vi "Should Read Body.vi"(8 "error in (no error)":errorcluster, 11 "Request in":refnum<class "Request.lvclass">) -> (0 "error out":errorcluster, 2 "Read Body?":bool, 3 "Request out":refnum<class "Request.lvclass">)   [LabVIEW 2023, in "Request.lvclass"]
doc: "Determines whether or not the Request should read a body, based on the Headers from the Client."
uses:
  Request.lvclass
  Request.lvclass/Request.ctl
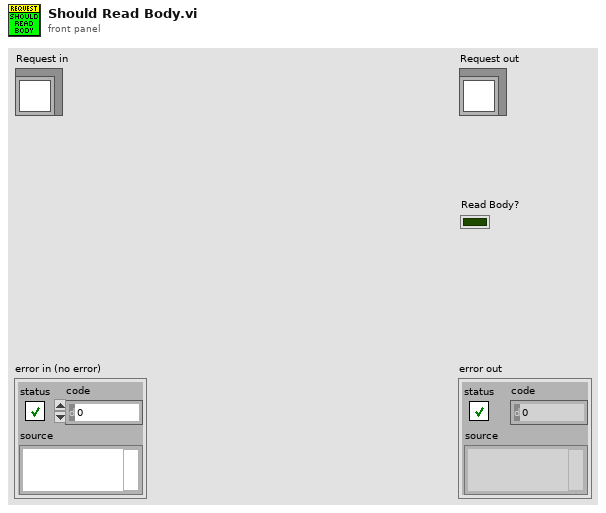
[diagram p1: front panel]
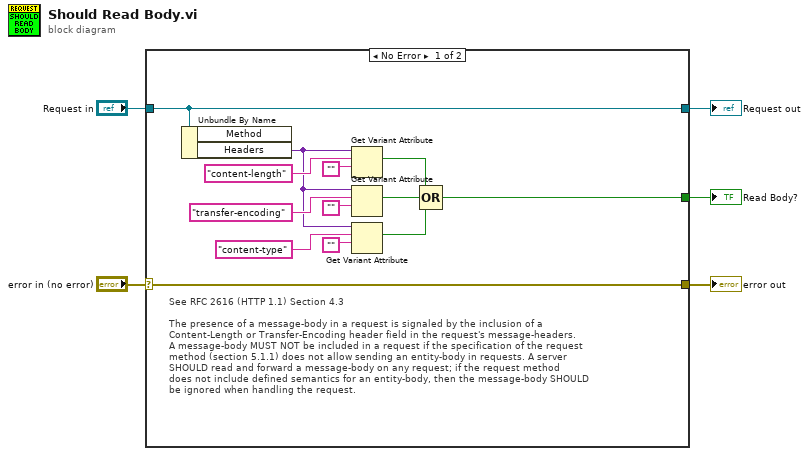
[diagram p0: block diagram]
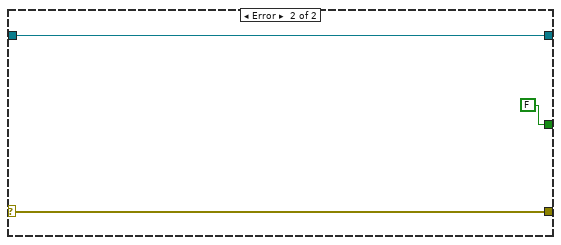
[diagram p2: hidden frame]
diagram:
  n1 = case shown="No Error" "error in (no error)" {
    selector: "error in (no error)" -> [w18 w21]
    tunnel: [w18 w21] -> w4
    tunnel: [w17 w20] -> w2
    tunnel: "Request in" -> [w17 w20]
    tunnel: [w11 FALSE] -> w1
    frame No Error {
      # "See RFC 2616 (HTTP 1.1) Section 4.3\n\nThe presence of a message-body in a request is signaled by the inclusion of a \nContent-Length or Transfer-Encoding header field in the request's message-headers. \nA message-body MUST NOT be included in a request if the specification of the request \nmethod (section 5.1.1) does not allow sending an entity-body in requests. A server \nSHOULD read and forward a message-body on any request; if the request method \ndoes not include defined semantics for an entity-body, then the message-body SHOULD \nbe ignored when handling the request."
      n2 = Unbundle By Name(w17) -> ("Headers"=w8:variant)  [unwired: 1 out]
      n3 = Get Variant Attribute(Variant=w8, name="content-length", default value (empty Variant)="") -> (found=w12:bool)  [unwired: 1 in, 3 out]
      n4 = Get Variant Attribute(Variant=w8, name="transfer-encoding", default value (empty Variant)="") -> (found=w7:bool)  [unwired: 1 in, 3 out]
      n5 = Get Variant Attribute(Variant=w8, name="content-type", default value (empty Variant)="") -> (found=w6:bool)  [unwired: 1 in, 3 out]
      n6 = Compound Arithmetic op=OR(w12, w7, w6) -> (w11:bool)
    }
    frame Error {
    }
  }
  "error out" <- w4
  "Request out" <- w2
  "Read Body?" <- w1
